vi "Write Analog_Output.vi"(10 "Analog_Output.lvclass":refnum<class "Analog_Output.lvclass">, 11 "Experiment in":refnum<class "Experiment.lvclass">) -> (3 "Experiment out":refnum<class "Experiment.lvclass">)   [LabVIEW 2013]
uses:
  Experiment.lvclass
  Analog_output/Analog_Output.lvclass
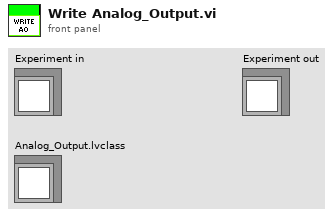
[diagram p1: front panel]
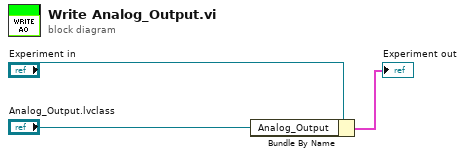
[diagram p0: block diagram]
diagram:
  n1 = Bundle By Name(cluster="Experiment in", "Analog_Output"="Analog_Output.lvclass") -> (→"Experiment out":cluster{})
